vi "3Axis_Acel_v2.vi"(9 "Roll_A":dbl, 10 "Yaw_A":dbl, 11 "Pitch_A":dbl) -> (0 "RAH":u8, 1 "YAL":u8, 2 "YAH":u8, 3 "PAL":u8, 4 "RAL":u8, 5 "PAH":u8)   [LabVIEW 2017]
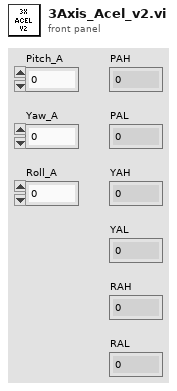
[diagram p1: front panel]
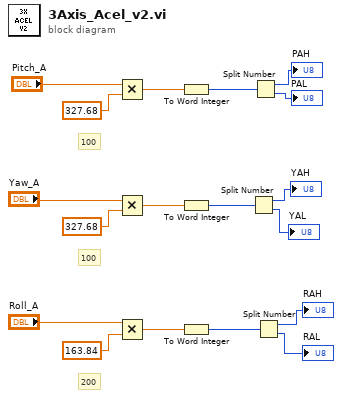
[diagram p0: block diagram]
diagram:
  # "200"
  # "100"
  # "100"
  n1 = Multiply(x="Pitch_A", y=327.68) -> (x*y=w10:dbl)
  n2 = Multiply(x="Yaw_A", y=327.68) -> (x*y=w8:dbl)
  n3 = Multiply(x="Roll_A", y=163.84) -> (x*y=w3:dbl)
  n4 = To Word Integer(number=w10) -> (16bit integer=w9:i16)
  n5 = To Word Integer(number=w8) -> (16bit integer=w5:i16)
  n6 = To Word Integer(number=w3) -> (16bit integer=w2:i16)
  n7 = Split Number(x=w5) -> (hi(x)=→"YAH":u8, lo(x)=→"YAL":u8)
  n8 = Split Number(x=w9) -> (hi(x)=→"PAH":u8, lo(x)=→"PAL":u8)
  n9 = Split Number(x=w2) -> (hi(x)=→"RAH":u8, lo(x)=→"RAL":u8)
